vi "Close UDP AND TCP connections.vi"(4 "error in":errorcluster, 6 "appended array 2":refnum<vi>[](array[refnum]), 7 "appended array":variant[](array[variant])) -> ()   [LabVIEW 2020]
panel:
  out "Array":refnum<k5>[](array[refnum])
  out "error out":errorcluster
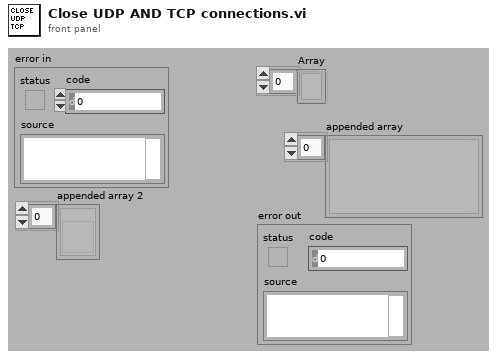
[diagram p1: front panel]
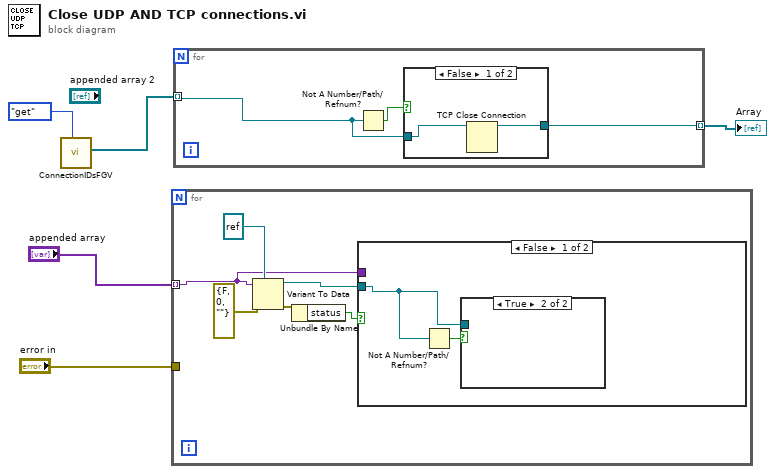
[diagram p0: block diagram]
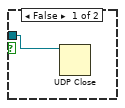
[diagram p3: hidden frame]
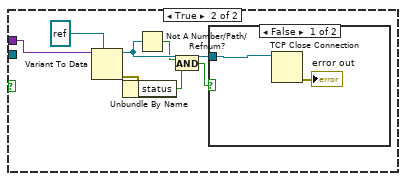
[diagram p4: hidden frame]
diagram:
  n1 = call "ConnectionIDsFGV.vi"("Command"=enum16{"add", "get", "init"}."get") -> ("ID Array"=w1:refnum<k5>[])  [unwired: 10 in]
  n2 = for {
    tunnel: "appended array" -> [w6] mode=indexing
    tunnel: "error in" -> [_]
    n3 = Variant To Data(error in=errorcluster {"status"=FALSE, "code"=0, "source"=""}, type=refnum<k16> refnum ("connection ID"), Variant=w6) -> (data=w7:refnum<k16>, error out=w9:errorcluster)
    n4 = Unbundle By Name(w9) -> ("status"=w8:bool)
    n5 = case shown="False" w8 {
      tunnel: w7 -> [w12 _]
      tunnel: w6 -> [_ w21]
      frame False {
        n6 = Not A Number/Path/Refnum?(number/path/refnum=w12) -> (NaN/Path/Refnum?=w13:bool)
        n7 = case shown="True" w13 {
          tunnel: w12 -> [w14 _]
          frame False {
            n8 = UDP Close(connection ID=w14) -> ()  [unwired: 1 in, 2 out]
          }
          frame True {
          }
        }
      }
      frame True {
        n9 = Variant To Data(type=refnum<k5> refnum ("connection ID"), Variant=w21) -> (data=w18:refnum<k5>, error out=w19:errorcluster)  [unwired: 1 in]
        n10 = Unbundle By Name(w19) -> ("status"=w17:bool)
        n11 = Not A Number/Path/Refnum?(number/path/refnum=w18) -> (NaN/Path/Refnum?=w16:bool)
        n12 = And(x=w16, y=w17) -> (x .and. y?=w15:bool)
        n13 = case shown="False" w15 {
          tunnel: w18 -> [w23 _]
          frame False {
            n14 = TCP Close Connection(connection ID=w23) -> (error out=→"error out":errorcluster)  [unwired: 2 in, 1 out]
          }
          frame True {
          }
        }
      }
    }
  }
  n15 = for {
    tunnel: w1 -> [w24] mode=indexing
    tunnel: [w25] -> w3 mode=indexing
    n16 = Not A Number/Path/Refnum?(number/path/refnum=w24) -> (NaN/Path/Refnum?=w26:bool)
    n17 = case shown="False" w26 {
      tunnel: w24 -> [w28 w29]
      tunnel: [w27 w29] -> w25
      frame False {
        n18 = TCP Close Connection(connection ID=w28) -> (connection ID out=w27:refnum<k5>)  [unwired: 2 in, 1 out]
      }
      frame True {
      }
    }
  }
  "Array" <- w3
